vi "Write Oscilloscope.vi"(8 "error in (no error)":errorcluster caption="entrée d'erreur (pas d'erreur)", 10 "Oscilloscope.lvclass":refnum<class "Oscilloscope.lvclass">, 11 "Control-Server en entrée":refnum<class "Control-Server.lvclass">) -> (0 "error out":errorcluster caption="sortie d'erreur", 3 "Control-Server en sortie":refnum<class "Control-Server.lvclass">)   [LabVIEW 2020, in "Control-Server.lvclass"]
uses:
  Control-Server.lvclass
  Oscilloscope/Oscilloscope.lvclass
  Control-Server.lvclass/Control-Server.ctl
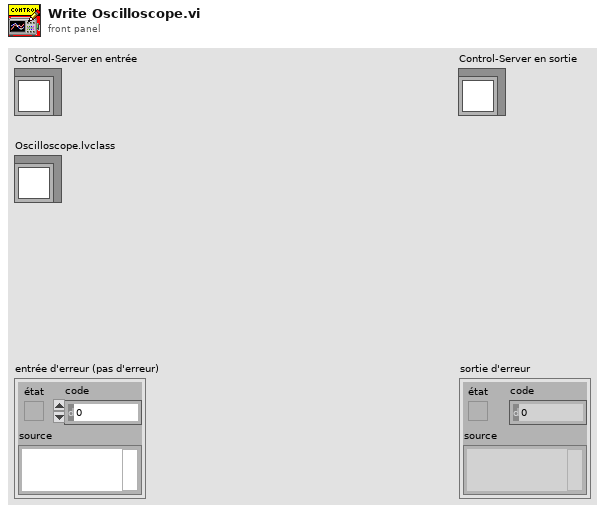
[diagram p1: front panel]
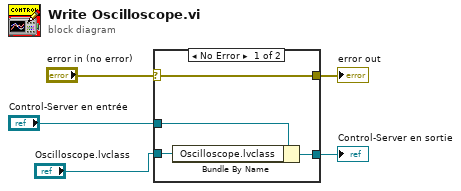
[diagram p0: block diagram]
diagram:
  n1 = case shown="No Error" "error in (no error)" {
    selector: "error in (no error)" -> [w9 w10]
    tunnel: [w9 w10] -> w4
    tunnel: [w7 w11] -> w2
    tunnel: "Control-Server en entrée" -> [w8 w11]
    tunnel: "Oscilloscope.lvclass" -> [w6 _]
    frame No Error {
      n2 = Bundle By Name(cluster=w8, "Oscilloscope.lvclass"=w6) -> (w7:refnum<class "Control-Server.lvclass">)
    }
    frame Error {
    }
  }
  "error out" <- w4
  "Control-Server en sortie" <- w2
